vi "Get Active Measurements.vi"(8 "error in (no error)":errorcluster {"code" format="%.0x"}, 9 "ValBufferSize":i32=2048, 10 "Channel":string, 11 "instrument handle":refnum<k15>) -> (0 "error out":errorcluster {"code" format="%.0x"}, 1 "ValActualSize":i32, 2 "Val":i32[](array[numeric]), 3 "instrument handle out":refnum<k15>)   [LabVIEW 2014, in "Agilent NA.lvlib"]
doc: "Get the active measurement in the channel"
uses:
  Agilent NA.lvlib
  AgNA.dll
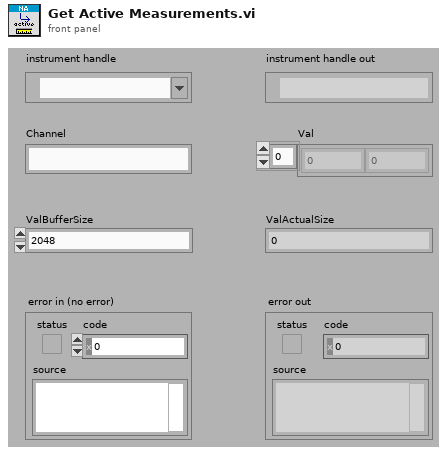
[diagram p1: front panel]
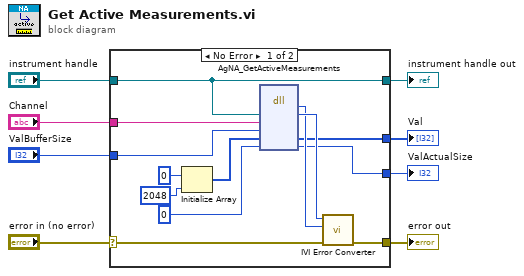
[diagram p0: block diagram]
diagram:
  n1 = case shown="No Error" "error in (no error)" {
    selector: "error in (no error)" -> [w19 w23]
    tunnel: [w18 w23] -> w8
    tunnel: "Channel" -> [w17 _]
    tunnel: [w14 _] -> w5
    tunnel: [w12 _] -> w4
    tunnel: [w11 w22] -> w3
    tunnel: "instrument handle" -> [w11 w22]
    tunnel: "ValBufferSize" -> [w9 _]
    frame No Error {
      n2 = Initialize Array(0 ("element"), 2048 ("dimension size")) -> (w16:i32[])
      n3 = dll-call lib="AgNA**.dll" fn="AgNA_GetActiveMeasurements"("Vi"=w11, "Channel"=w17, "ValBufferSize"=w9, "Val"=w16, "ValActualSize"=0) -> (w20:i32, "Vi"=w21:u32, "Val"=w14:i32[], "ValActualSize"=w12:i32)  [unwired: 5 in, 2 out]
      n4 = call "IVI Error Converter.vi"("error in (no error)"=w19, "IVI error code (0)"=w20, "instrument handle"=w21) -> ("error out"=w18:errorcluster)  [unwired: 7 in, 1 out]
    }
    frame Error {
    }
  }
  "error out" <- w8
  "instrument handle out" <- w3
  "Val" <- w5
  "ValActualSize" <- w4
